vi "读取参数.vi"(0 "Slave ID":u8=10, 1 "starting address":u16, 2 "quantity":u16, 3 "Error in":errorcluster caption="Error in (no error)") -> (7 "values":u16[](array[numeric]), 10 "error out":errorcluster)   [LabVIEW 2016, in "质控单元.lvlib"]
uses:
  <vilib>/Plasmionique/MB Master/MB_Master_Serial/MB_Master_Serial.lvclass
  F:/Program Files/National Instruments/LabVIEW 2016/vi.lib/Plasmionique/MB Master/MB_Master/MB_Master.lvclass
  <vilib>/Plasmionique/MB Master/MB Master.lvlib
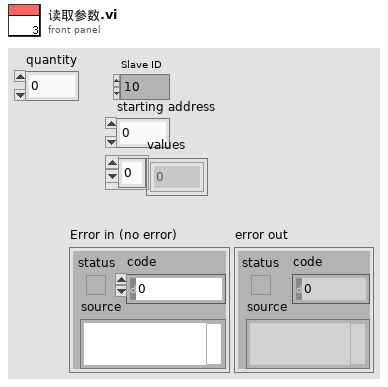
[diagram p1: front panel]
types:
  T1 = cluster{"baud rate (bps)":u32, "stop bits":u16, "parity":u16, "flow control":u16, "timeout":u32, "retries":i32}
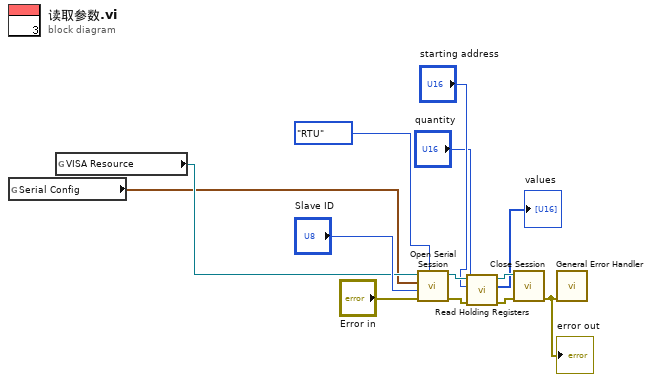
[diagram p0: block diagram]
diagram:
  n1 = global read "串口参数全局.vi" "Serial Config"() -> (w8:T1)
  n2 = global read "串口参数全局.vi" "VISA Resource"() -> (w9:refnum<visa-resource-name>)
  n3 = call <vilib>:"Open Serial Session.vi"("Mode (RTU)"=enum16{"RTU", "ASCII"}."RTU", "Error in"="Error in", "Slave ID"="Slave ID", "Serial Config"=w8, "VISA Resource"=w9) -> ("Error out"=w6:errorcluster, "MB_Serial session"=w7:refnum<class "MB_Master_Serial.lvclass">)  [unwired: 5 in]
  n4 = call <vilib>:"Read Holding Registers.vi"("error in (no error)"=w6, "quantity"="quantity", "starting address"="starting address", "MB session in"=w7) -> ("error out"=w4:errorcluster, "Registers"=→"values":u16[], "MB session out"=w5:refnum<class "MB_Master_Serial.lvclass">)  [unwired: 5 in]
  n5 = call-dynamic "Close Session.vi"("error in (no error)"=w4, "MB_Serial session"=w5) -> ("error out"=w11:errorcluster)  [unwired: 9 in]
  "error out" <- w11
  n6 = call <vilib>:"General Error Handler.vi"("error in (no error)"=w11) -> ()  [unwired: 10 in, 5 out]
